vi "Tetra_Atten.vi"(0 "COMPORT":refnum<visa-resource-name>="COM4", 3 "RevC(T)":bool=TRUE, 5 "error in (no error)":errorcluster, 6 "Open Ser(t)":bool, 7 "TxAtten(num)":i32 min=0 max=3 step=1, 8 "Close Ser(t)":bool, 9 "Atten(dB)":dbl min=0.0 max=31.5 step=0.5, 11 "RO(t)":bool) -> (10 "txatten(name)":string="5 - 8", 12 "atten(value)":dbl, 14 "comport":refnum<visa-resource-name>="COM4", 16 "atten(code)ary (ro)":i32[](array[numeric])=[0, 5, 5, 63], 19 "error out":errorcluster)   [LabVIEW 2018]
panel:
  out "Success":bool=TRUE
  out "concatenated string":string="txatten \r\n0)   atten0: 0\r\n1)   atten1: 5\r\n2)   atten2: 5\r\n3)   atten3: 63\r\n>"
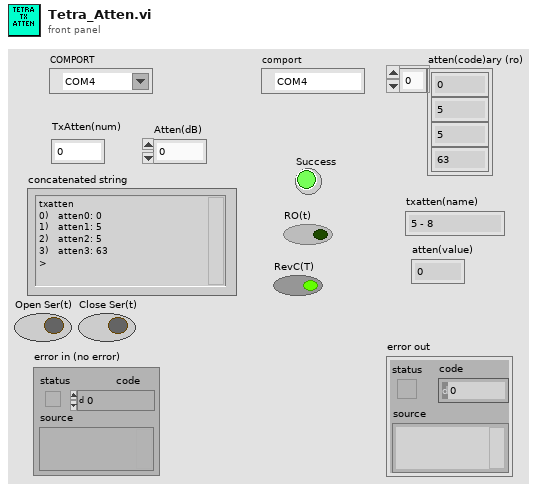
[diagram p1: front panel]
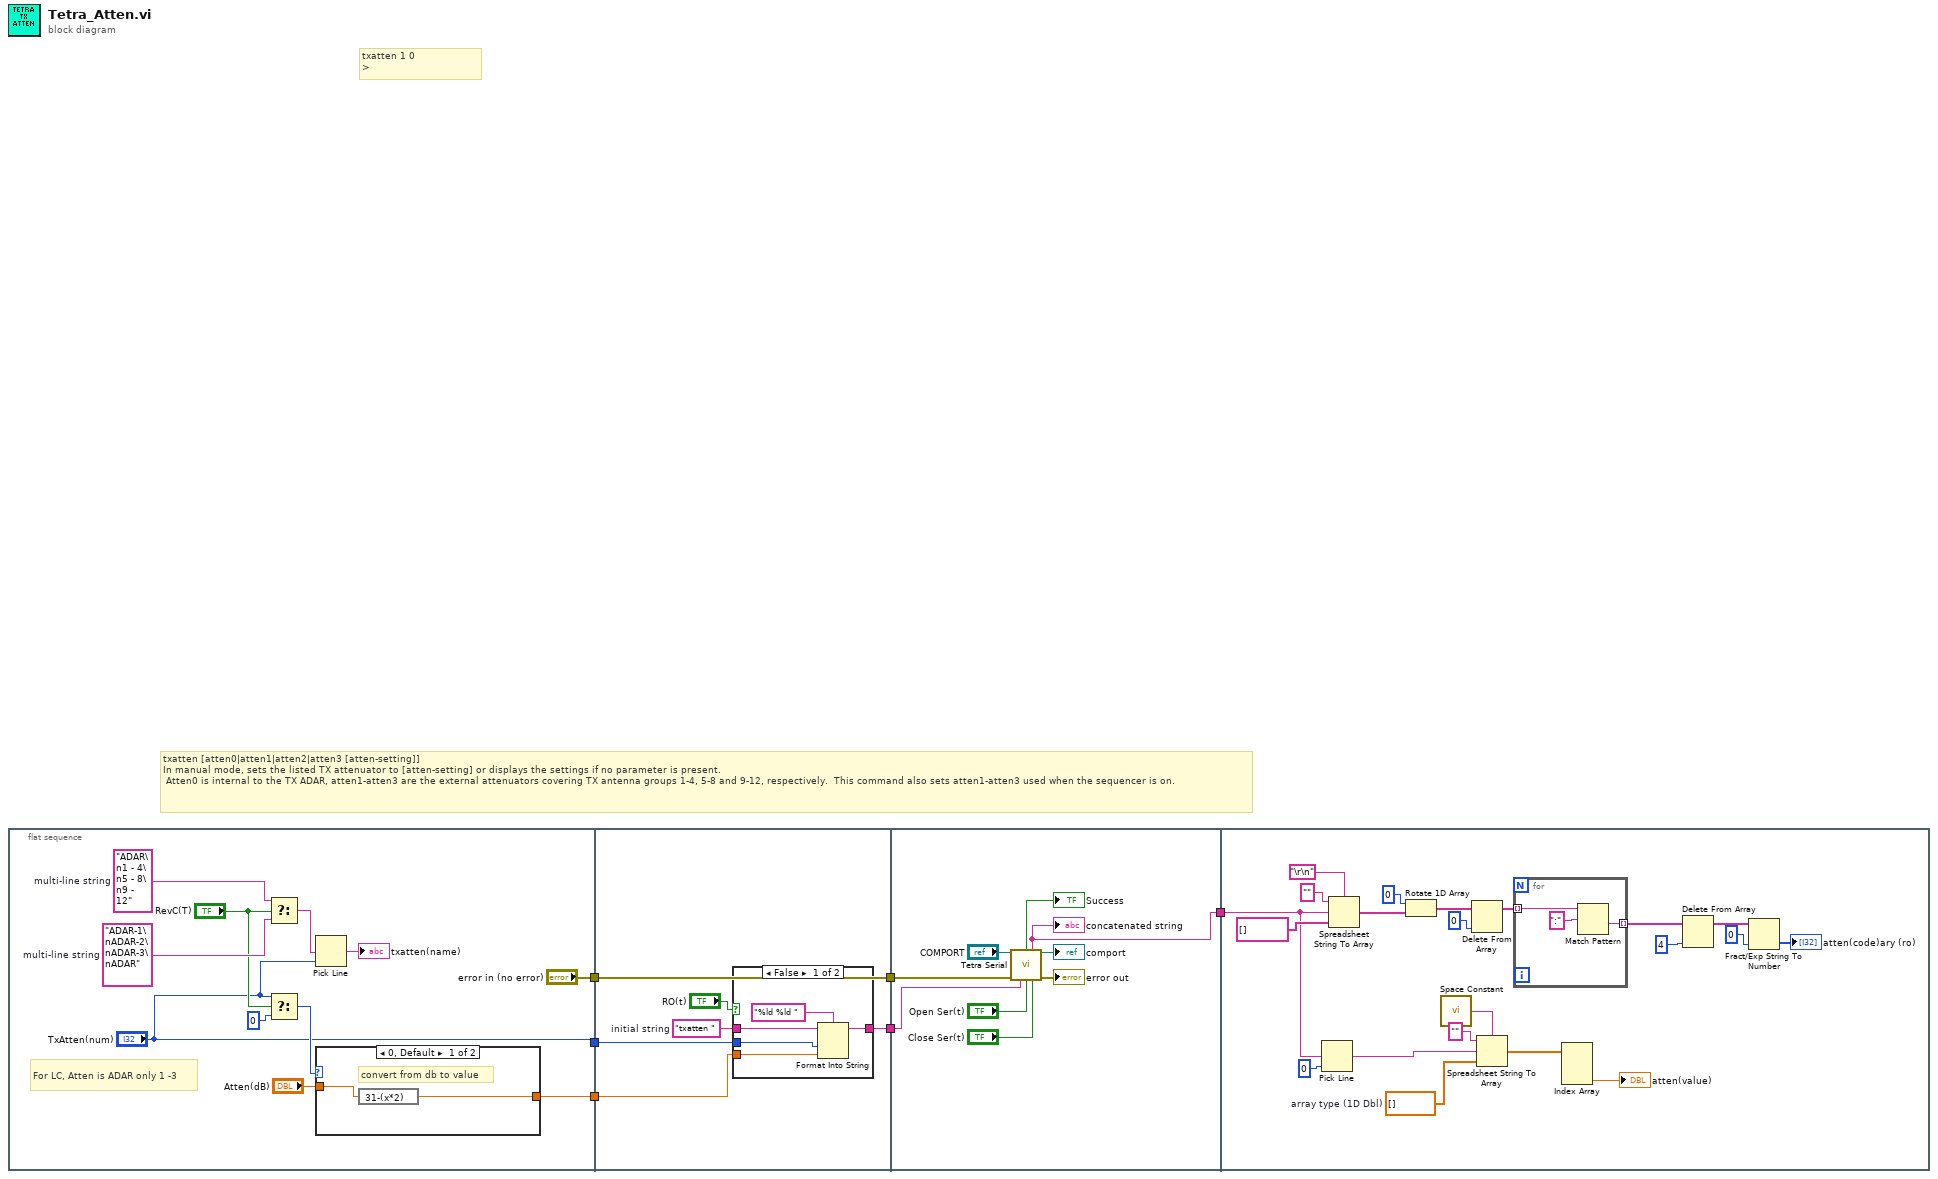
[diagram p0: block diagram]
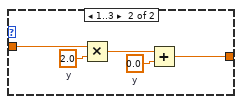
[diagram p2: hidden frame]
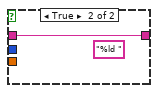
[diagram p3: hidden frame]
diagram:
  # "txatten [atten0|atten1|atten2|atten3 [atten-setting]]\nIn manual mode, sets the listed TX attenuator to [atten-setting] or displays the settings if no parameter is present. \n Atten0 is internal to the TX ADAR, atten1-atten3 are the external attenuators covering TX antenna groups 1-4, 5-8 and 9-12, respectively.  This command also sets atten1-atten3 used when the sequencer is on."
  # "txatten 1 0\n>"
  n1 = flat-sequence {
    tunnel: [w15] -> w6
    tunnel: ["error in (no error)"] -> w5
    tunnel: ["TxAtten(num)"] -> w1
    tunnel: w6 -> [w27]
    tunnel: w5 -> [w25]
    tunnel: [w26] -> w4
    tunnel: [w25] -> w3
    tunnel: w1 -> [w28]
    tunnel: w4 -> [w38]
    tunnel: w3 -> [w39]
    tunnel: [w37] -> w2
    tunnel: w2 -> [w46]
    frame #0 {
      w11 = "ADAR-1\nADAR-2\nADAR-3\nADAR"  # multi-line string
      w13 = "ADAR\n1 - 4\n5 - 8\n9 - 12"  # multi-line string
      # "For LC, Atten is ADAR only 1 -3"
      n2 = Select(t=w13, s="RevC(T)", f=w11) -> (s? t:f=w12:string)
      n3 = Select(t="TxAtten(num)", s="RevC(T)", f=0) -> (s? t:f=w10:i32)
      n4 = Pick Line(multi-line string=w12, line index="TxAtten(num)") -> (output string=→"txatten(name)":string)  [unwired: 1 in]
      n5 = case shown="0, Default" w10 {
        tunnel: "Atten(dB)" -> [w19 w24]
        tunnel: [w18 w20] -> w15
        frame 0, Default {
          # "convert from db to value"
          n6 = expression code="31-(x*2)"(w19) -> (w18:dbl)
        }
        frame 1..3 {
          w21 = 0.0  # y
          w23 = 2.0  # y
          n7 = Multiply(x=w24, y=w23) -> (x*y=w22:dbl)
          n8 = Add(x=w22, y=w21) -> (x+y=w20:dbl)
        }
      }
    }
    frame #1 {
      w29 = "txatten "  # initial string
      n9 = case shown="False" "RO(t)" {
        tunnel: [w35 w36] -> w26
        tunnel: w29 -> [w34 w36]
        tunnel: w28 -> [w33 _]
        tunnel: w27 -> [w32 _]
        frame False {
          n10 = Format Into String(format string="%ld %ld ", initial string=w34, w33, w32) -> (resulting string=w35:string)  [unwired: 1 in, 1 out]
        }
        frame True {
          (unwired) "%ld "
        }
      }
    }
    frame #2 {
      n11 = call "Tetra Serial.vi"("COMPORT"="COMPORT", "error in (no error)"=w39, "Command"=w38, "Open Ser(t)"="Open Ser(t)", "Close Ser(t)"="Close Ser(t)") -> ("Success"=→"Success":bool, "output"=w37:string, "comport"=→"comport":refnum<visa-resource-name>, "error out"=→"error out":errorcluster)  [unwired: 6 in, 1 out]
      "concatenated string" <- w37
    }
    frame #3 {
      w49 = dbl[] []  # array type (1D Dbl)
      n12 = Pick Line(multi-line string=w46, line index=0) -> (output string=w57:string)  [unwired: 1 in]
      n13 = Spreadsheet String To Array(delimiter (Tab)="\r\n", format string="", spreadsheet string=w46, array type (2D Dbl)=string[] []) -> (array=w61:string[])
      n14 = Rotate 1D Array(1:w61, 2:0 ("n")) -> (0:w62:string[])
      n15 = call <vilib>:"Space Constant.vi"() -> ("String"=w58:string)
      n16 = Delete From Array(array=w62, index=0) -> (array with subset deleted=w63:string[])  [unwired: 1 in, 1 out]
      n17 = Spreadsheet String To Array(delimiter (Tab)=w58, format string="", spreadsheet string=w57, array type (2D Dbl)=w49) -> (array=w59:dbl[])
      n18 = for {
        tunnel: w63 -> [w69] mode=indexing
        tunnel: [w67] -> w64 mode=indexing
        n19 = Match Pattern(string=w69, regular expression=":") -> (after substring=w67:string)  [unwired: 1 in, 3 out]
      }
      n20 = Index Array(array=w59) -> (element #3=→"atten(value)":dbl)  [unwired: 3 in, 2 out]
      n21 = Delete From Array(array=w64, index=4) -> (array with subset deleted=w65:string[])  [unwired: 1 in, 1 out]
      n22 = Fract/Exp String To Number(string=w65, default (0 dbl)=0 ("default (0 DBL)")) -> (number=→"atten(code)ary (ro)":i32[])  [unwired: 2 in, 1 out]
    }
  }
